vi "Keithley_apply.vi"(6 "Level":dbl, 7 "Meas. CH Type":T2 items=["Current", "Voltage", "IV"], 8 "Channel (Channel A)":T3, 9 "Input CH Type":T1 items=["Current", "Voltage", ""], 10 "Node Out in":string, 11 "VISA Refnum in":refnum<visa-resource-name>) -> (0 "Output":string, 2 "Node Out out":string, 3 "VISA Refnum out":refnum<visa-resource-name>)   [LabVIEW 2012]
uses:
  Keithley 2600 Series/Keithley 2600 Series.lvlib
  Keithley 2600 Series/Public/Channel.ctl
  controls/MeasurementType.ctl
  controls/KeithlyChannelType.ctl
panel:
  in  "error in (no error)":errorcluster
  out "error out":errorcluster
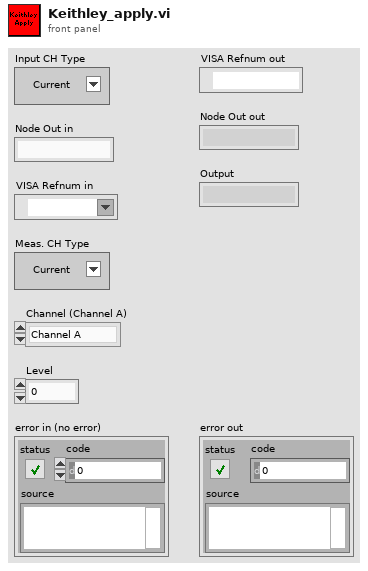
[diagram p1: front panel]
types:
  T1 = typedef "KeithlyChannelType.ctl" = u16
  T2 = typedef "MeasurementType.ctl" = u16
  T3 = typedef "Keithley 2600 Series.lvlib/Channel.ctl" = enum32{"Channel A", "Channel B"}
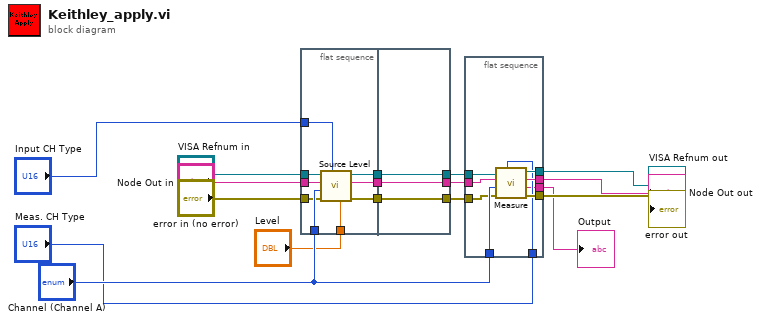
[diagram p0: block diagram]
diagram:
  n1 = flat-sequence {
    tunnel: "Channel (Channel A)" -> [w26]
    tunnel: "Input CH Type" -> [w25]
    tunnel: "error in (no error)" -> [w24]
    tunnel: "Node Out in" -> [w23]
    tunnel: "VISA Refnum in" -> [w22]
    tunnel: "Level" -> [w18]
    tunnel: [w21] -> w3
    tunnel: [w20] -> w2
    tunnel: [w19] -> w1
    tunnel: [w27] -> w6
    tunnel: [w28] -> w7
    tunnel: [w29] -> w8
    tunnel: w3 -> [w29]
    tunnel: w2 -> [w28]
    tunnel: w1 -> [w27]
    frame #0 {
      n2 = call "Source Level.vi"("Level (0.000)"=w18, "Function (Current)"=w25, "error in (no error)"=w24, "Channel (Channel A)"=w26, "Node In"=w23, "VISA resource name"=w22) -> ("error out"=w21:errorcluster, "Node Out"=w20:string, "VISA resource name out"=w19:refnum<visa-resource-name>)  [unwired: 3 out]
    }
    frame #1 {
    }
  }
  n3 = flat-sequence {
    tunnel: "Channel (Channel A)" -> [w38]
    tunnel: [w37] -> w16
    tunnel: [w36] -> w15
    tunnel: [w35] -> w14
    tunnel: "Meas. CH Type" -> [w34]
    tunnel: w8 -> [w33]
    tunnel: w7 -> [w32]
    tunnel: w6 -> [w31]
    tunnel: [w30] -> w4
    frame #0 {
      n4 = call "Measure.vi"("Function (Current)"=w34, "error in (no error)"=w33, "Channel (Channel A)"=w38, "Node In"=w32, "VISA resource name"=w31) -> ("error out"=w37:errorcluster, "Output"=w30:string, "Node Out"=w36:string, "VISA resource name out"=w35:refnum<visa-resource-name>)  [unwired: 2 in, 1 out]
    }
  }
  "error out" <- w16
  "Node Out out" <- w15
  "VISA Refnum out" <- w14
  "Output" <- w4
